vi "Seq File Is Valid.vi"(8 "error in (no error)":errorcluster, 11 "Seq File Path":string) -> (0 "error out":errorcluster)   [LabVIEW 2014, in "teststand-api.lvlib" / "teststand-api.lvclass"]
uses:
  teststand-api.lvclass
  <vilib>/Utility/error.llb/Error Cluster From Error Code.vi
  <vilib>/ErrorRing/Error Ring.xnode
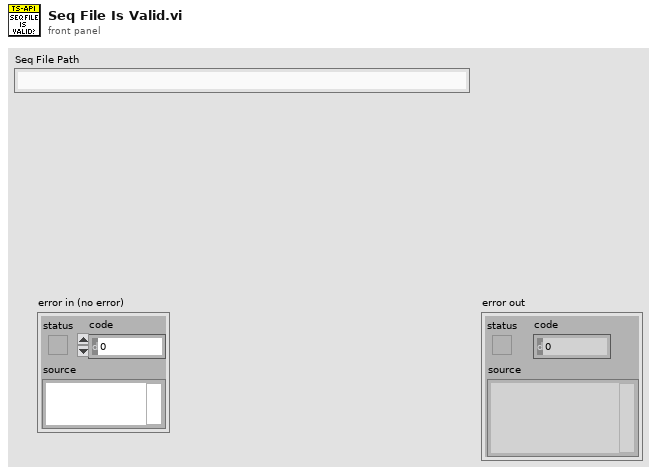
[diagram p1: front panel]
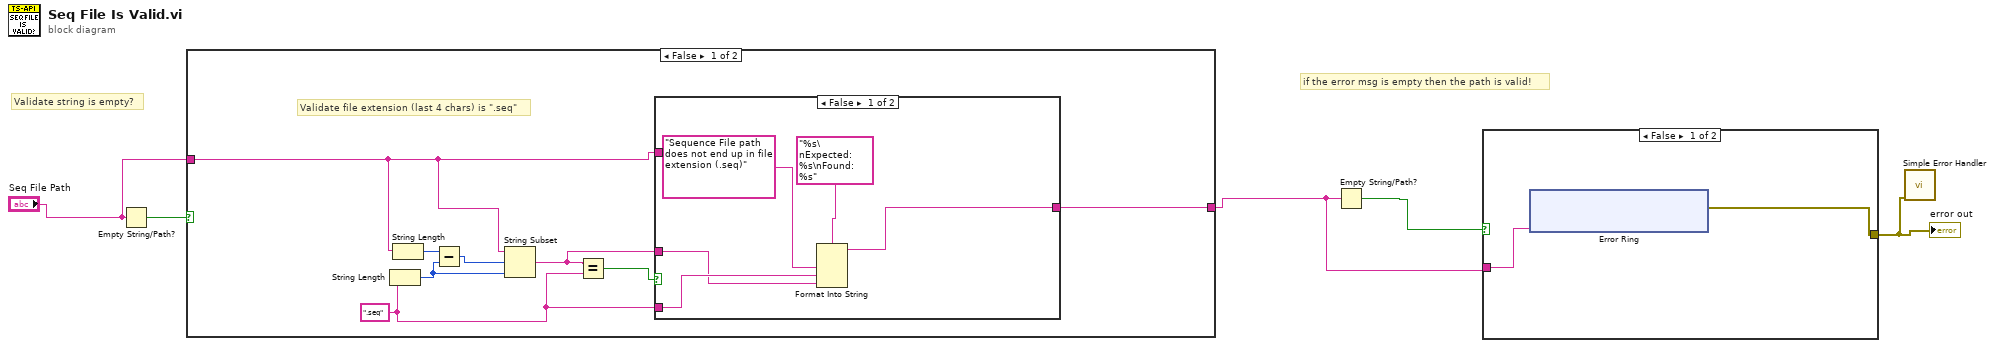
[diagram p0: block diagram]
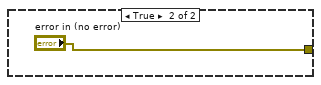
[diagram p2: hidden frame]
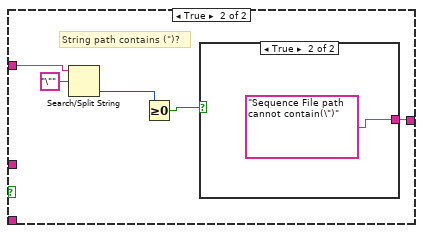
[diagram p3: hidden frame]
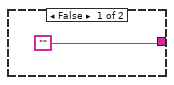
[diagram p4: hidden frame]
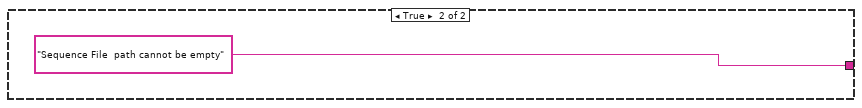
[diagram p5: hidden frame]
diagram:
  # "if the error msg is empty then the path is valid!"
  # "Validate string is empty?"
  n1 = Empty String/Path?(string/path="Seq File Path") -> (empty?=w5:bool)
  n2 = case shown="False" w5 {
    tunnel: "Seq File Path" -> [w6 _]
    tunnel: [w7 "Sequence File  path cannot be empty"] -> w1
    frame False {
      w9 = ".seq" ("search string")
      # "Validate file extension (last 4 chars) is \".seq\""
      n3 = String Length(string=w9) -> (length=w11:i32)
      n4 = String Length(string=w6) -> (length=w13:i32)
      n5 = Subtract(x=w13, y=w11) -> (x-y=w12:i32)
      n6 = String Subset(string=w6, offset (0)=w12, length (rest)=w11) -> (substring=w8:string)
      n7 = Equal?(x=w8, y=w9) -> (x = y?=w10:bool)
      n8 = case shown="False" w10 {
        tunnel: [w16 w19] -> w7
        tunnel: w9 -> [w15 _]
        tunnel: w8 -> [w14 _]
        tunnel: w6 -> [_ w23]
        frame False {
          n9 = Format Into String(format string="%s\nExpected: %s\nFound: %s", "Sequence File path does not end up in file extension (.seq)", w15, w14) -> (resulting string=w16:string)  [unwired: 2 in, 1 out]
        }
        frame True {
          # "String path contains (\")?"
          n10 = Search/Split String(string=w23, search string/char (-)="\"") -> (offset of match=w21:i32)  [unwired: 1 in, 2 out]
          n11 = Greater Or Equal To 0?(x=w21) -> (x >= 0?=w20:bool)
          n12 = case shown="True" w20 {
            tunnel: ["" "Sequence File path cannot contain(\")"] -> w19
            frame False {
            }
            frame True {
            }
          }
        }
      }
    }
    frame True {
    }
  }
  n13 = Empty String/Path?(string/path=w1) -> (empty?=w3:bool)
  n14 = case shown="False" w3 {
    tunnel: [w27 "error in (no error)"] -> w2
    tunnel: w1 -> [w28 _]
    frame False {
      n15 = xnode "Error Ring"("parameter 0"=w28) -> ("error out"=w27:errorcluster)
    }
    frame True {
    }
  }
  "error out" <- w2
  n16 = call <vilib>:"Simple Error Handler.vi"("error in (no error)"=w2) -> ()  [unwired: 4 in, 5 out]
